vi "DotNet-多探头启动器.vi"(11 "数值输入控件":u16=1) -> (0 "输出簇":T1, 1 "面板vi引用[]":refnum<vi>[](array[refnum]), 2 "中间启动者VI引用":refnum<vi>, 3 "错误输出":errorcluster)   [LabVIEW 2017]
uses:
  8b769e95-7625-417b-9e30-421626132829.vi
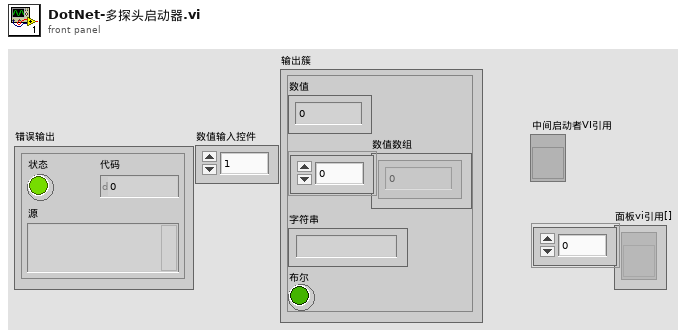
[diagram p1: front panel]
types:
  T1 = cluster{"数值":i32, "数值数组":i32[], "字符串":string, "布尔":bool}
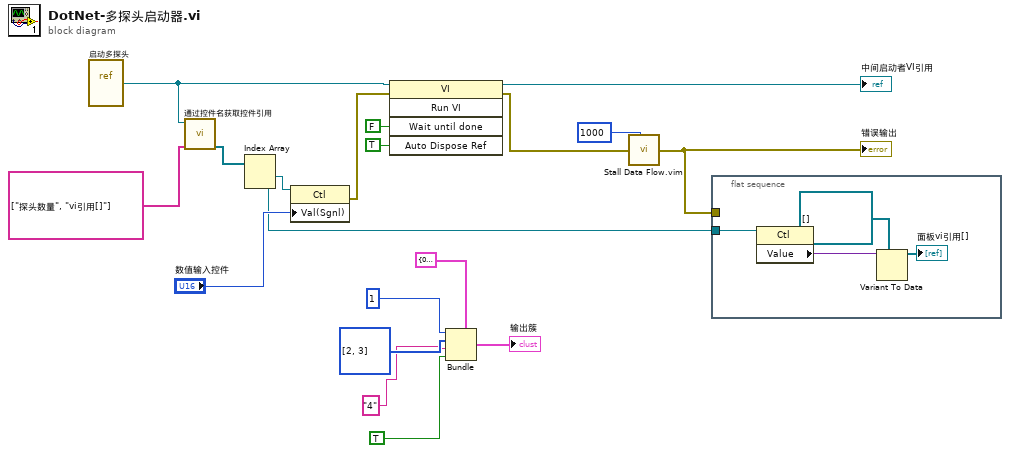
[diagram p0: block diagram]
diagram:
  n1 = vi-ref "启动多探头.vi"() -> (w15:refnum<vi>)
  n2 = call "通过控件名获取控件引用.vi"("控件名数组"=string[] ["探头数量", "vi引用[]"], "VI引用"=w15) -> ("控件引用输出"=w16:refnum<vi>[])  [unwired: 7 in, 2 out]
  n3 = Index Array(array=w16) -> (element #1=w13:refnum<vi>, element #2=w2:refnum<vi>)  [unwired: 2 in]
  n4 = property class="Ctl"(reference=w13, "Val(Sgnl)"="数值输入控件") -> (error out=w11:errorcluster)  [unwired: 1 in, 1 out]
  n5 = invoke class="VI" method="Run VI"(reference=w15, error in=w11, "Wait until done"=FALSE ("结束前等待"), "Auto Dispose Ref"=TRUE ("自动销毁引用")) -> (reference out=→"中间启动者VI引用":refnum<vi>, error out=w17:errorcluster)  [unwired: 1 in, 3 out]
  n6 = Bundle(cluster=T1 {"数值"=0, "数值数组"=[], "字符串"="", "布尔"=FALSE} ("簇"), "数值"=1, "数值数组"=i32[] [2, 3], "字符串"="4", "布尔"=TRUE) -> (→"输出簇":T1)
  n7 = call "Stall Data Flow.vim"("value in"=w17, "milliseconds to wait"=u32 1000) -> ("value out"=w1:errorcluster)  [unwired: 1 out]
  "错误输出" <- w1
  n8 = flat-sequence {
    tunnel: w2 -> [w23]
    tunnel: w1 -> [_]
    frame #0 {
      n9 = property class="Ctl"(reference=w23) -> ("Value"=w22:variant)  [unwired: 1 in, 2 out]
      n10 = Variant To Data(type=refnum<vi>[] [] ("vi引用[]"), Variant=w22) -> (data=→"面板vi引用[]":refnum<vi>[])  [unwired: 1 in, 1 out]
    }
  }
